vi "rethinkdb_msg_base64_encode.vi"(11 "string":string) -> (3 "base64":string)   [LabVIEW 2017]
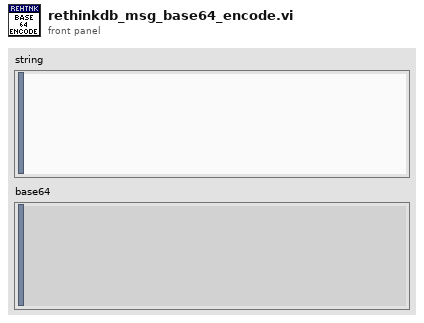
[diagram p1: front panel]
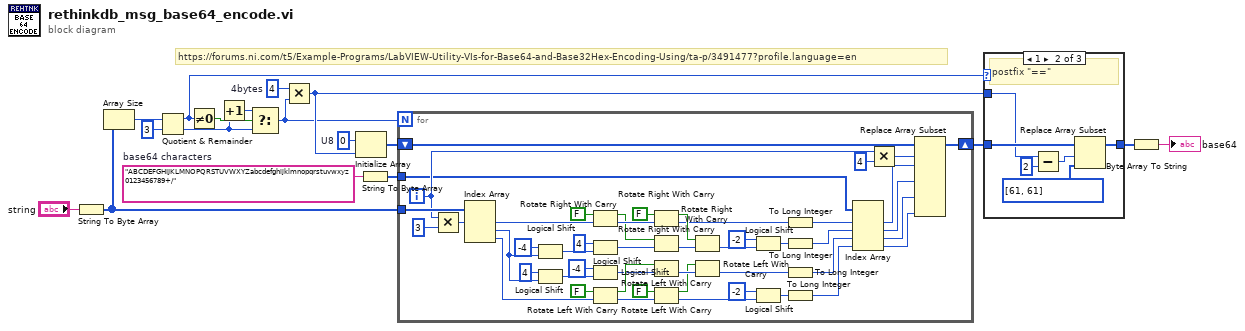
[diagram p0: block diagram]
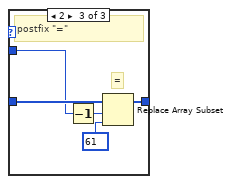
[diagram p3: hidden frame]
diagram:
  w2 = "ABCDEFGHIJKLMNOPQRSTUVWXYZabcdefghijklmnopqrstuvwxyz0123456789+/"  # base64 characters
  w15 = 4  # 4bytes
  w17 = u8 0  # U8
  # "https://forums.ni.com/t5/Example-Programs/LabVIEW-Utility-VIs-for-Base64-and-Base32Hex-Encoding-Using/ta-p/3491477?profile.language=en"
  n1 = String To Byte Array(string="string") -> (unsigned byte array=w9:u8[])
  n2 = Array Size(array=w9) -> (size(s)=w8:i32)
  n3 = Quotient & Remainder(x=w8, y=3) -> (x-y*floor(x/y)=w14:i32, floor(x/y)=w4:i32)
  n4 = Not Equal To 0?(x=w14) -> (x != 0?=w13:bool)
  n5 = Increment(x=w4) -> (x+1=w5:i32)
  n6 = Select(t=w5, s=w13, f=w4) -> (s? t:f=w3:i32)
  n7 = Multiply(x=w15, y=w3) -> (x*y=w10:i32)
  n8 = Initialize Array(w17, w10) -> (w16:u8[])
  n9 = String To Byte Array(string=w2) -> (unsigned byte array=w1:u8[])
  n10 = for {
    N: w3 -> [_]
    shift-right: [w65] -> w12
    shift-left: w16 -> [w66]
    tunnel: w9 -> [w27]
    tunnel: w1 -> [w19]
    i -> [w21]
    n11 = Multiply(x=w21, y=3) -> (x*y=w23:i32)
    n12 = Index Array(array=w27, index #1=w23) -> (element #1=w26:u8, element #2=w25:u8, element #3=w24:u8)  [unwired: 2 in]
    n13 = Logical Shift(y=i16 -4, x=w25) -> (x << y=w32:u8)
    n14 = Logical Shift(y=i16 4, x=w25) -> (x << y=w35:u8)
    n15 = Rotate Right With Carry(2:w26, 3:FALSE ("carry")) -> (0:w61:u8, 1:w60:bool)
    n16 = Logical Shift(y=i16 4, x=w32) -> (x << y=w30:u8)
    n17 = Logical Shift(y=i16 -4, x=w35) -> (x << y=w33:u8)
    n18 = Rotate Left With Carry(2:w24, 3:FALSE ("carry")) -> (0:w54:u8, 1:w51:bool)
    n19 = Rotate Right With Carry(2:w61, 3:FALSE ("carry")) -> (0:w42:u8, 1:w59:bool)
    n20 = Rotate Right With Carry(2:w30, 3:w60) -> (0:w58:u8)  [unwired: 1 out]
    n21 = Rotate Left With Carry(2:w33, 3:w51) -> (0:w49:u8)  [unwired: 1 out]
    n22 = Rotate Left With Carry(2:w54, 3:FALSE ("carry")) -> (0:w53:u8, 1:w28:bool)
    n23 = Rotate Right With Carry(2:w58, 3:w59) -> (0:w57:u8)  [unwired: 1 out]
    n24 = Rotate Left With Carry(2:w49, 3:w28) -> (0:w47:u8)  [unwired: 1 out]
    n25 = Logical Shift(y=i16 -2, x=w57) -> (x << y=w43:u8)
    n26 = Logical Shift(y=i16 -2, x=w53) -> (x << y=w48:u8)
    n27 = To Long Integer(number=w42) -> (32bit integer=w41:i32)
    n28 = To Long Integer(number=w43) -> (32bit integer=w44:i32)
    n29 = To Long Integer(number=w47) -> (32bit integer=w45:i32)
    n30 = To Long Integer(number=w48) -> (32bit integer=w46:i32)
    n31 = Index Array(array=w19, index #1=w41, index #2=w44, index #3=w45, index #4=w46) -> (element #1=w40:u8, element #2=w39:u8, element #3=w38:u8, element #4=w37:u8)
    n32 = Multiply(x=w21, y=4) -> (x*y=w20:i32)
    n33 = Replace Array Subset(array=w66, new element #1=w40, index #1=w20, new element #2=w39, new element #3=w38, new element #4=w37) -> (w65:u8[])  [unwired: 3 in]
  }
  n34 = case shown="1" w14 {
    tunnel: w12 -> [w67 w70 w78]
    tunnel: [w67 w71 w75] -> w11
    tunnel: w10 -> [_ w69 w74]
    frame Default {
      # "no remainder"
    }
    frame 1 {
      # "postfix \"==\""
      n35 = Subtract(x=w69, y=2) -> (x-y=w72:i32)
      n36 = Replace Array Subset(array=w70, new element=u8[] [61, 61] ("new element/subarray"), index=w72) -> (w71:u8[])
    }
    frame 2 {
      # "="
      # "postfix \"=\""
      n37 = Decrement(x=w74) -> (x-1=w77:i32)
      n38 = Replace Array Subset(array=w78, new element=u8 61, index=w77) -> (w75:u8[])
    }
  }
  n39 = Byte Array To String(unsigned byte array=w11) -> (string=→"base64":string)
